vi "Untitled 1.vi"() -> ()   [LabVIEW 2014]
uses:
  U:/Visual Studio 2015/Projects/Exemple/Exemple/bin/Debug/Exemple.dll
  bin/Debug/Exemple.dll
panel:
  in  "Stop Button":bool
  in  "Blank Button":bool
  in  "String":string
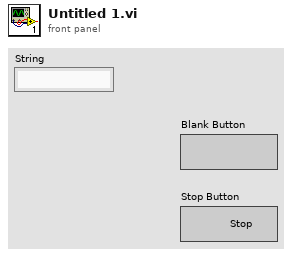
[diagram p1: front panel]
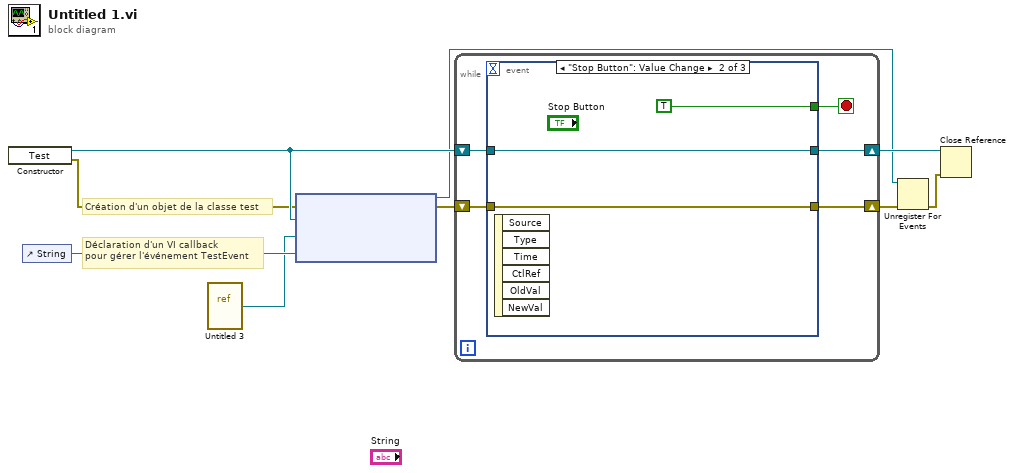
[diagram p0: block diagram]
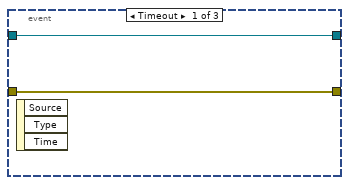
[diagram p2: hidden frame]
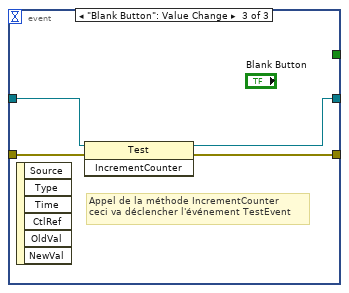
[diagram p3: hidden frame]
diagram:
  # "Déclaration d'un VI callback\npour gérer l'événement TestEvent"
  # "Création d'un objet de la classe test"
  n1 = constructor class="Test"() -> (reference out=w7:refnum<k24>, error out=w2:errorcluster)  [unwired: 3 in, 1 out]
  n2 = control-ref of="String"() -> (w9:refnum<vi>)
  n3 = vi-ref "Untitled 3.vi"() -> ("vi reference"=w8:refnum<vi>)
  n4 = node(w2, w7, w8, w9) -> (w5:refnum<k27>, w3:errorcluster)  [unwired: 1 in]
  n5 = while {
    shift-right: [w12] -> w6
    shift-left: w7 -> [w14]
    shift-right: [w11] -> w4
    shift-left: w3 -> [w10]
    stop <- w13 stop-if-true
    n6 = event shown="[1] \"Stop Button\": Value Change" {
      selector: _ -> [_ _ _]
      dyn-events: _ -> [_ _ _]
      timeout: _ -> [_ _ _]
      tunnel: w14 -> [w16 w18 w23]
      tunnel: [_ TRUE _] -> w13
      tunnel: [w16 w18 w22] -> w12
      tunnel: [w15 w17 w21] -> w11
      tunnel: w10 -> [w15 w17 w20]
      event Timeout {
        n7 = event-data() -> ()  [unwired: 1 in, 3 out]
      }
      event "Stop Button": Value Change {
        n8 = event-data() -> ()  [unwired: 1 in, 6 out]
      }
      event "Blank Button": Value Change {
        # "Appel de la méthode IncrementCounter\nceci va déclencher l'événement TestEvent"
        n9 = event-data() -> ()  [unwired: 1 in, 6 out]
        n10 = invoke class="Test" method="IncrementCounter"(reference=w23, error in=w20) -> (reference out=w22:refnum<k24>, error out=w21:errorcluster)  [unwired: 1 in, 1 out]
      }
    }
  }
  n11 = Unregister For Events(event registration refnum=w5, error in=w4) -> (error out=w1:errorcluster)
  n12 = Close Reference(reference=w6, error in (no error)=w1) -> ()  [unwired: 1 out]
